vi "Legend of All Colormaps.vi"() -> ()   [LabVIEW 2019]
uses:
  LV Colormap Names.ctl
  f871708b-1f91-45df-a74b-debef35ac716.vi
  1d75663b-af70-4854-a513-be56e357ce6c.vi
panel:
  out "Colormaps":T1(array[cluster])
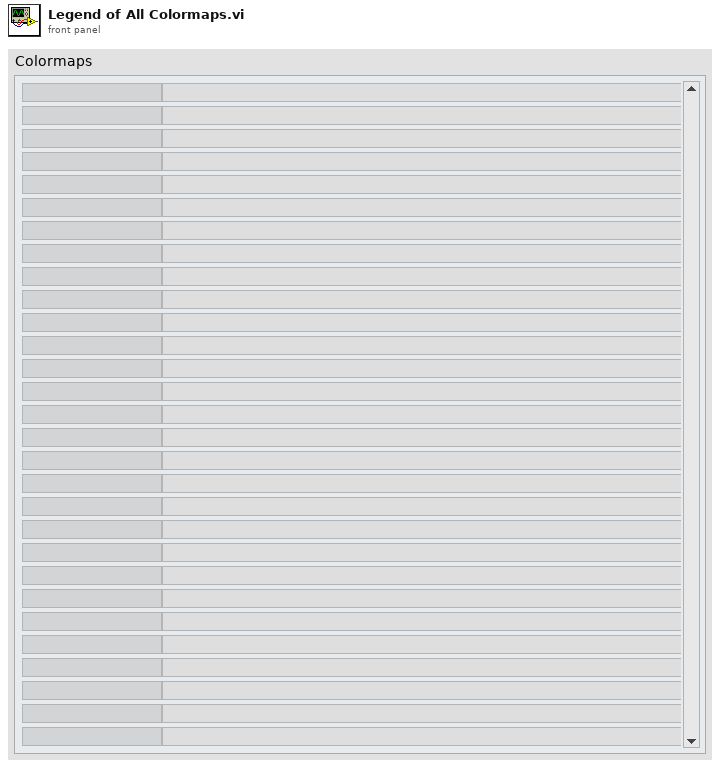
[diagram p1: front panel]
types:
  T1 = cluster{"Colormap Name":string, "2D Picture":picture}[]
  T2 = cluster{"Width":u16, "Style":enum32{"Solid", "Dash", "Dot", "DashDot", "DashDotDot"}}
  T3 = typedef "LV Colormap Names.ctl" = enum16{"Accent", "Accent_r", "Blues", "Blues_r", "BrBG", "BrBG_r", "BuGn", "BuGn_r", "BuPu", "BuPu_r", "CMRmap", "CMRmap_r", "Dark2", "Dark2_r", "GnBu", "GnBu_r", "Grays", "Grays_r", "Greens", "Greens_r", "Greys", "Greys_r", "OrRd", "OrRd_r", "Oranges", "Oranges_r", "PRGn", "PRGn_r", "Paired", "Paired_r", "Pastel1", "Pastel1_r", "Pastel2", "Pastel2_r", "PiYG", "PiYG_r", "PuBu", "PuBuGn", "PuBuGn_r", "PuBu_r", "PuOr", "PuOr_r", "PuRd", "PuRd_r", "Purples", "Purples_r", "RdBu", "RdBu_r", "RdGy", "RdGy_r", "RdPu", "RdPu_r", "RdYlBu", "RdYlBu_r", "RdYlGn", "RdYlGn_r", "Reds", "Reds_r", "Set1", "Set1_r", "Set2", "Set2_r", "Set3", "Set3_r", "Spectral", "Spectral_r", "Wistia", "Wistia_r", "YlGn", "YlGnBu", "YlGnBu_r", "YlGn_r", "YlOrBr", "YlOrBr_r", "YlOrRd", "YlOrRd_r", "afmhot", "afmhot_r", "autumn", "autumn_r", "berlin", "berlin_r", "binary", "binary_r", "bone", "bone_r", "brg", "brg_r", "bwr", "bwr_r", "cividis", "cividis_r", "cool", "cool_r", "coolwarm", "coolwarm_r", "copper", "copper_r", "cubehelix", "cubehelix_r", "flag", "flag_r", "gist_earth", "gist_earth_r", "gist_gray", "gist_gray_r", "gist_grey", "gist_grey_r", "gist_heat", "gist_heat_r", "gist_ncar", "gist_ncar_r", "gist_rainbow", "gist_rainbow_r", "gist_stern", "gist_stern_r", "gist_yarg", "gist_yarg_r", "gist_yerg", "gist_yerg_r", "gnuplot", "gnuplot2", "gnuplot2_r", "gnuplot_r", "gray", "gray_r", "grey", "grey_r", "hot", "hot_r", "hsv", "hsv_r", "inferno", "inferno_r", "jet", "jet_r", "magma", "magma_r", "managua", "managua_r", "nipy_spectral", "nipy_spectral_r", "ocean", "ocean_r", "pink", "pink_r", "plasma", "plasma_r", "prism", "prism_r", "rainbow", "rainbow_r", "seismic", "seismic_r", "spring", "spring_r", "summer", "summer_r", "tab10", "tab10_r", "tab20", "tab20_r", "tab20b", "tab20b_r", "tab20c", "tab20c_r", "terrain", "terrain_r", "turbo", "turbo_r", "twilight", "twilight_r", "twilight_shifted", "twilight_shifted_r", "vanimo", "vanimo_r", "viridis", "viridis_r", "winter", "winter_r"}
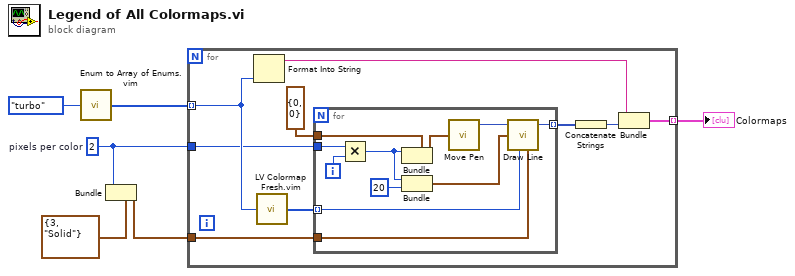
[diagram p0: block diagram]
diagram:
  w1 = u16 2  # pixels per color
  n1 = call "Enum to Array of Enums.vim"("enum"=LV_Colormap_Names."turbo" ("Colormap Name")) -> ("array of enums"=w5:T3[])
  n2 = Bundle(cluster=T2 {"Width"=3, "Style"=enum."Solid"} ("pen"), "Width"=w1) -> (w2:T2)  [unwired: 1 in]
  n3 = for {
    tunnel: w5 -> [w10] mode=indexing
    tunnel: w2 -> [w15]
    tunnel: [w11] -> w4 mode=indexing
    tunnel: w1 -> [w8]
    n4 = Format Into String(w10) -> (resulting string=w9:string)  [unwired: 3 in, 1 out]
    n5 = call "LV Colormap Fresh.vim"("Colormap Name"=w10) -> ("Colormap"=w14:u32[])  [unwired: 14 in]
    n6 = for {
      tunnel: [w26] -> w13 mode=indexing
      tunnel: cluster{"x":i16, "y":i16} {"x"=0, "y"=0} ("new position") -> [w24]
      tunnel: w15 -> [w22]
      tunnel: w14 -> [w18] mode=indexing
      tunnel: w8 -> [w16]
      i -> [w17]
      n7 = Multiply(x=w16, y=w17) -> (x*y=w21:i32)
      n8 = Bundle(cluster=w24, "x"=w21) -> (w23:cluster{"x":i16, "y":i16})  [unwired: 1 in]
      n9 = Bundle(w21, "y"=i16 20) -> (w19:cluster{i32, "y":i16})  [unwired: 1 in]
      n10 = call <vilib>:"Move Pen.vi"("new position"=w23) -> ("new picture"=w25:picture)  [unwired: 4 in]
      n11 = call <vilib>:"Draw Line.vi"("picture"=w25, "end point"=w19, "color(black)"=w18, "pen"=w22) -> ("new picture"=w26:picture)  [unwired: 5 in]
    }
    n12 = Concatenate Strings(w13) -> (w12:picture)
    n13 = Bundle(w9, w12) -> (w11:cluster{string, picture})  [unwired: 1 in]
  }
  "Colormaps" <- w4
